vi "DAQTest.vi"() -> ()   [LabVIEW 2018]
panel:
  out "data":dynamicdata(graph)
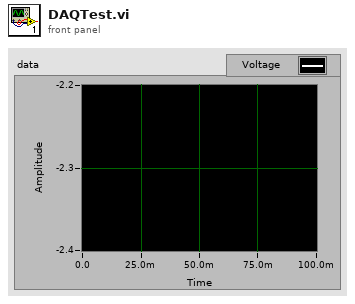
[diagram p1: front panel]
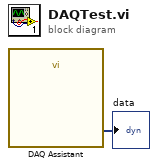
[diagram p0: block diagram]
diagram:
  n1 = call "DAQ Assistant"() -> ("data"=→"data":dynamicdata)  [unwired: 17 in, 2 out]
